vi "JY Mono Example.vi"() -> ()   [LabVIEW 2020]
doc: "This VI is an example on how to use the HORIBA Jobin Yvon Monochromator control VIs. To use this VI, press the Run button in LabVIEW.\n\nThe VI will retreive all configured monochromators from the computer's resgistry.\n\nSelect the desired monochromator from the Mono ID combo box and press the Connect button to start communications with that device. If the Force Initialization button is enabled, the monochromator will start its automatic calibration routine. If the Force Initialization button is not enabled, the sofwtare will keep the monochromator in its current positions.\n\nAfter connecting to the instrumnet, the VI will retreive the current positions of all movable motors in the system. This will continue until the Move To Target Position or Stop buttons are pressed.\n\nMove to Target Positions will move the monochromator to the postions entered in the indicators of the VI.\n\nStop will stop running the VI."
panel:
  out "Gratings":dbl[](array[numeric])=[1200.0, 300.0]
  in  "Target\nSide Exit":dbl
  in  "Target\nFront Exit":dbl
  in  "Target\nSide Entrance":dbl
  in  "Target\nFront Entrance":dbl
  in  "Exit Mirror":u16(ring)=2 caption="Target Position Exit Mirror" items=["Front"=2, "Side"=3]
  in  "Entrance Mirror":u16(ring)=2 caption="Target Position\nEntrance Mirror" items=["Front"=2, "Side"=3]
  out "error out":errorcluster
  in  "Target Grating":string(combo)="2"
  in  "Target WL":dbl=898.0
  in  "Move To\nTarget Positions":bool
  out "Units":string="nm"
  in  "Connect":bool
  out "Status":string="Initialized"
  out "Emulating":bool
  out "Initialized":bool=TRUE
  out "Current UniqueID":string="Mono4"
  in  "Force\nInitialization":bool
  in  "STOP":bool
  out "Units":string="mm"
  out "Units":string="mm"
  out "Units":string="mm"
  out "Units":string="mm"
  out "Side Exit":dbl
  out "Front Exit":dbl
  out "Side Entrance":dbl
  out "Front Entrance":dbl
  out "Exit Mirror\nPosition":i32(ring)=2 items=["EntranceMirror", "ExitMirror", "Front", "Side"]
  out "Entrance Mirror\nPosition":i32(ring)=2 items=["EntranceMirror", "ExitMirror", "Front", "Side"]
  out "Current Description":string="1" caption="Description"
  out "Grating Index":i32=1
  out "Current Grating":dbl=1200.0
  out "Current WL":dbl=897.9988
  in  "Mono ID":string(combo)="Mono4"
  # "Setup"
  # "Grating / Wavelength Control"
  # "Slits"
  # "Swing Mirrors"
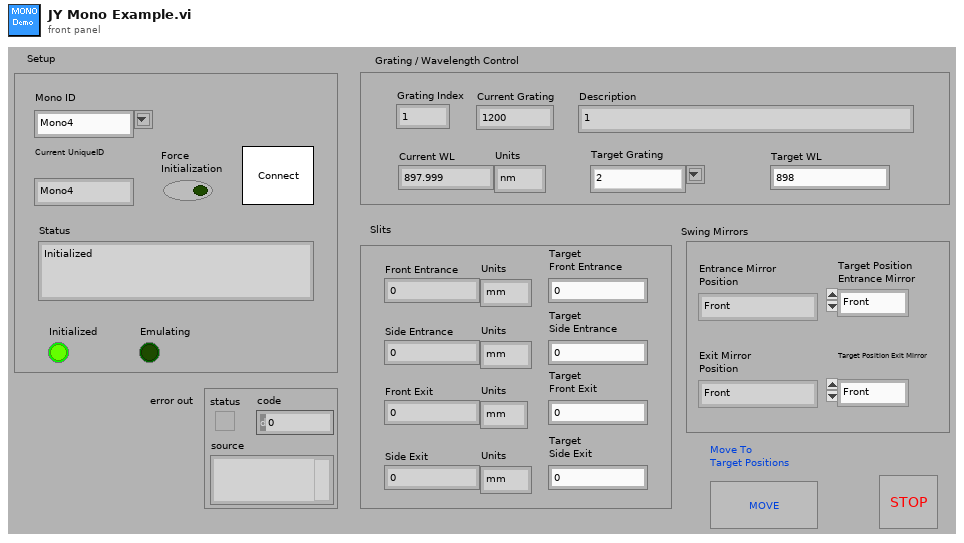
[diagram p1: front panel]
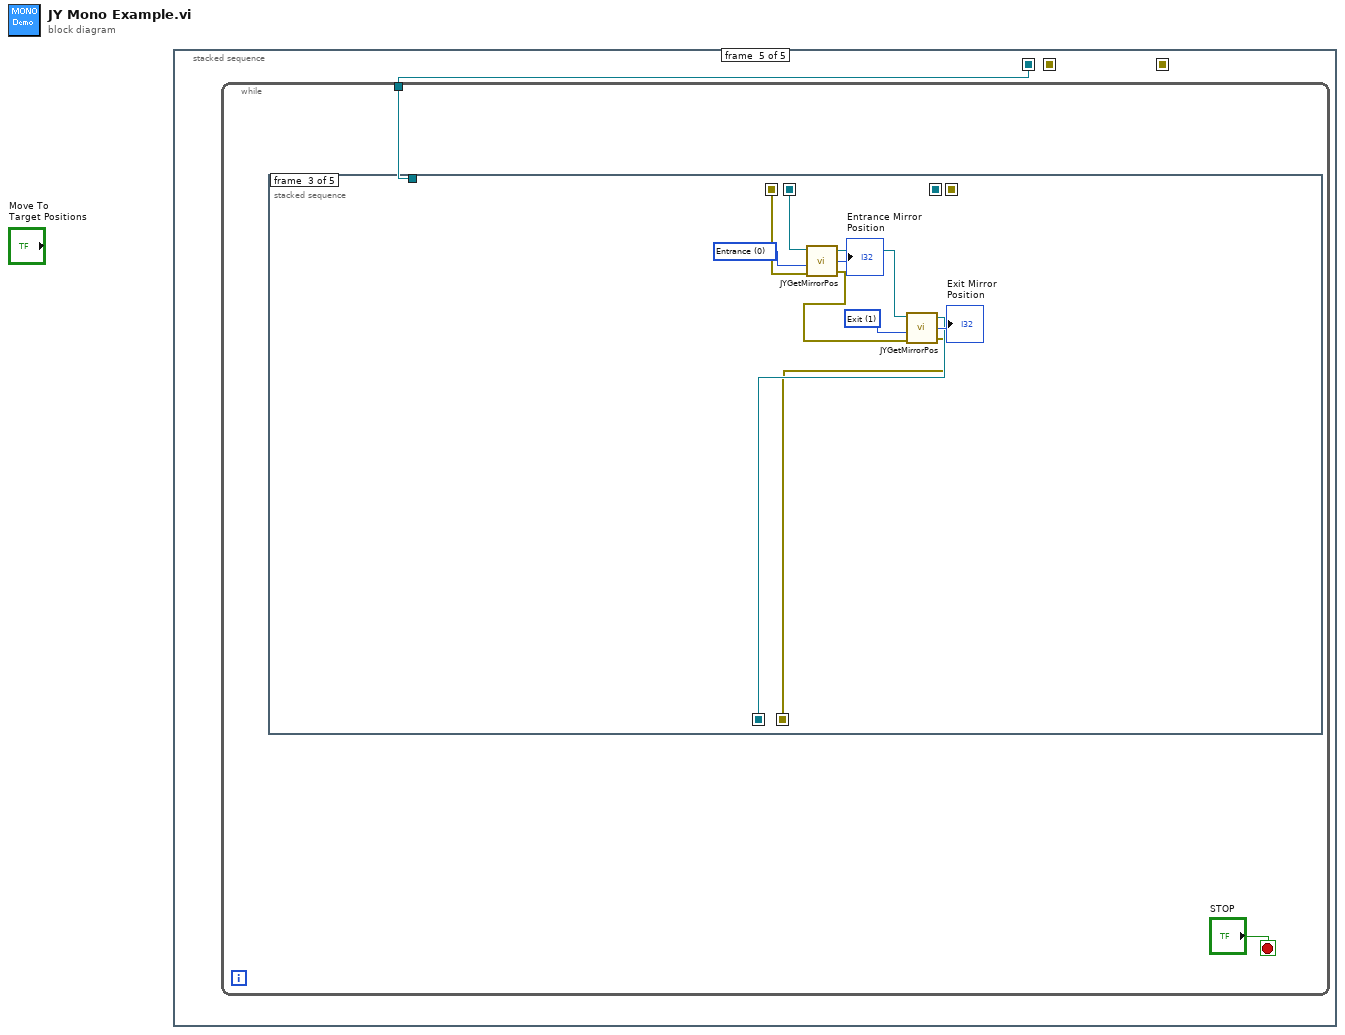
[diagram p0: block diagram]
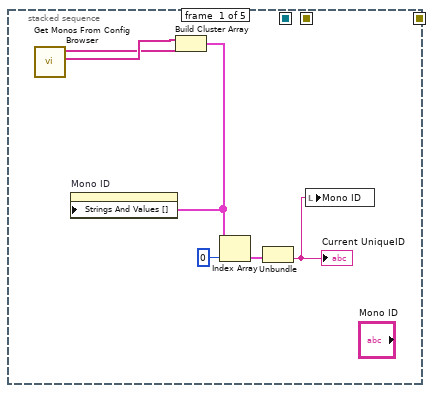
[diagram p2: hidden frame]
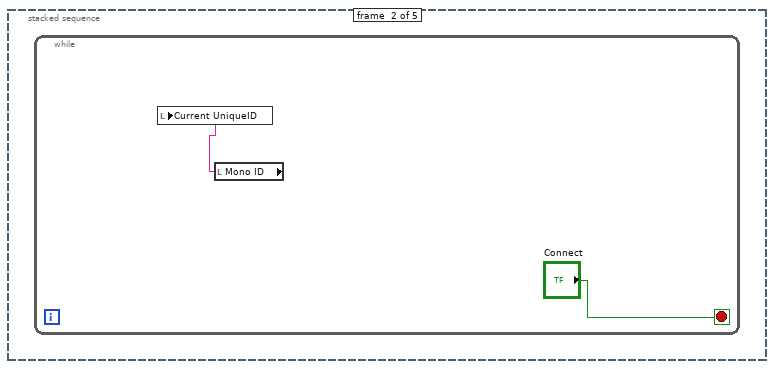
[diagram p3: hidden frame]
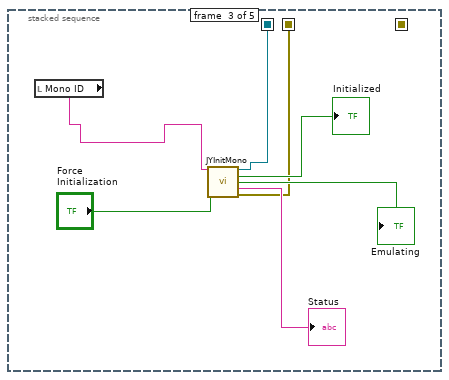
[diagram p4: hidden frame]
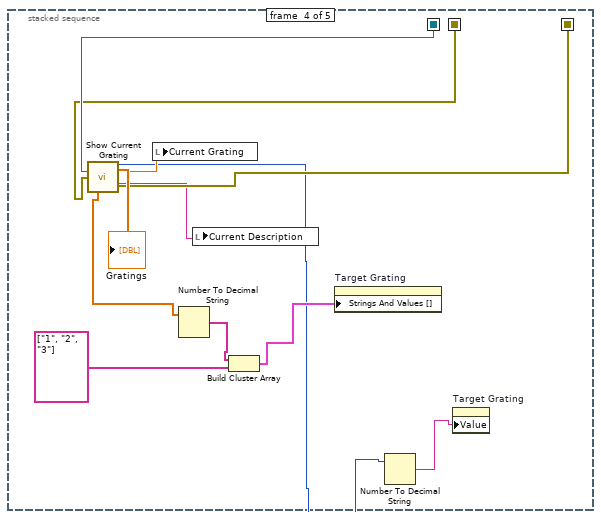
[diagram p5: hidden frame]
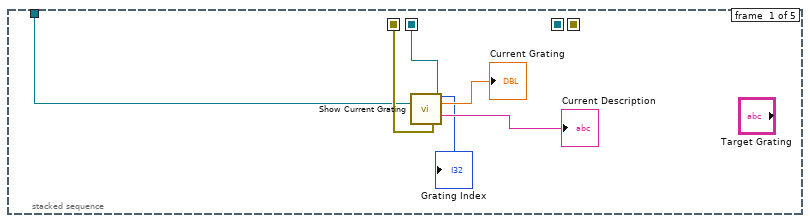
[diagram p6: hidden frame]
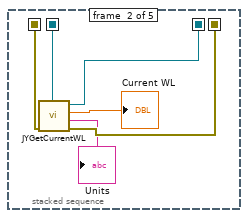
[diagram p7: hidden frame]
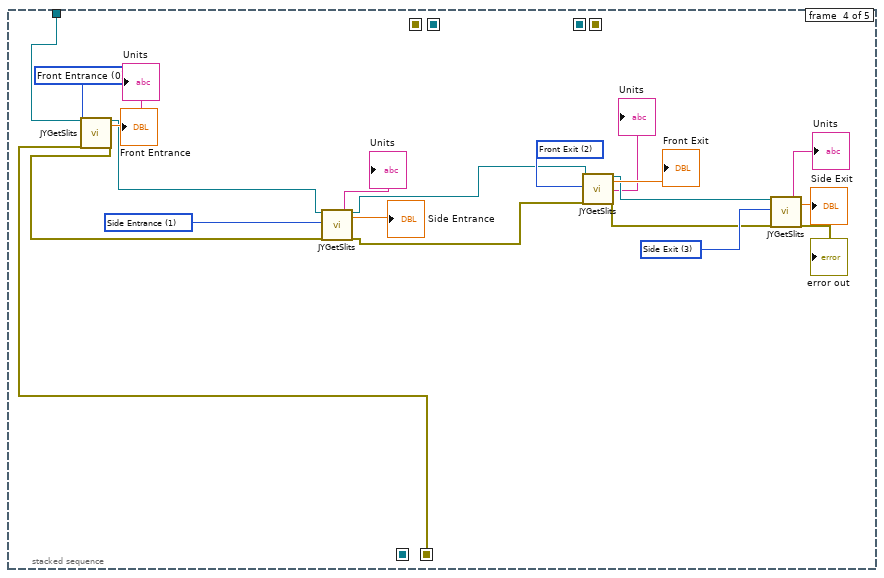
[diagram p8: hidden frame]
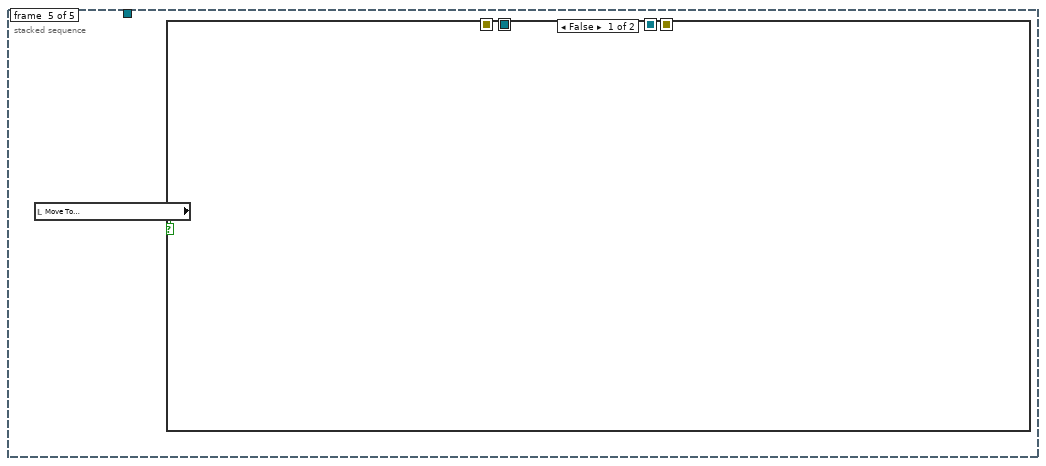
[diagram p9: hidden frame]
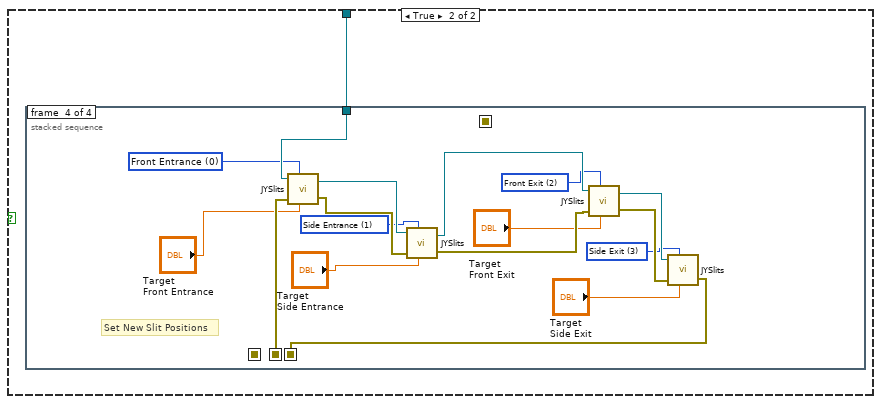
[diagram p10: hidden frame]
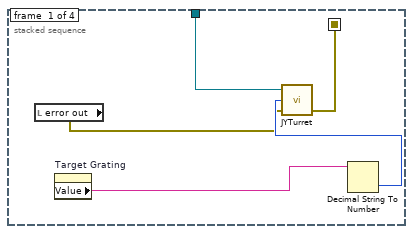
[diagram p11: hidden frame]
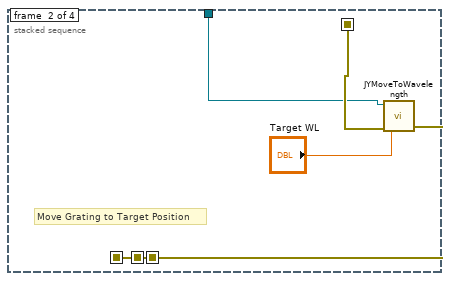
[diagram p12: hidden frame]
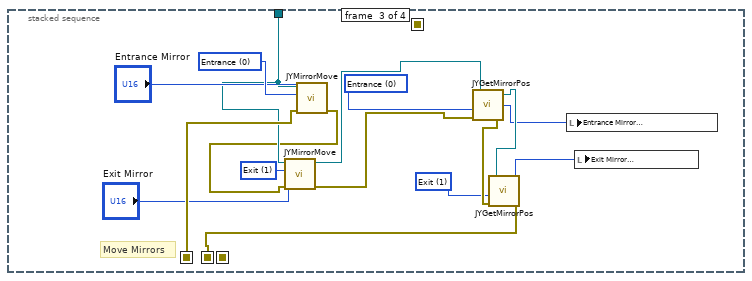
[diagram p13: hidden frame]
diagram:
  n1 = stacked-sequence {
    seq-local: [_ _ w10 _ _] -> [_ _ _ w22 w27]
    seq-local: [_ _ w9 _ _] -> [_ _ _ w21 _]
    seq-local: [_ _ _ w20 _] -> [_ _ _ _ _]
    frame #0 {
      n2 = call "Get Monos From Config Browser.vi"() -> ("UniqueIDs"=w5:string[], "Mono ID"=w6:string[])  [unwired: 3 in, 1 out]
      n3 = Build Cluster Array(w6, w5) -> (w3:cluster{"String":string, "String":string}[])
      n4 = property on="Mono ID" class="CmbBox"("Strings And Values []"=w3) -> ()  [unwired: 2 in, 2 out]
      n5 = Index Array(array=w3, index=0) -> (element=w4:cluster{"String":string, "String":string})
      n6 = Unbundle(w4) -> ("String"=w1:string)  [unwired: 1 out]
      "Current UniqueID" <- w1
      n7 = local write "Mono ID"(w1) -> ()
    }
    frame #1 {
      n8 = while {
        stop <- "Connect" stop-if-true
        n9 = local read "Mono ID"() -> (w7:string)
        n10 = local write "Current UniqueID"(w7) -> ()
      }
    }
    frame #2 {
      n11 = local read "Mono ID"() -> (w14:string)
      n12 = call "JYInitMono.vi"("Unique ID"=w14, "Force Init"="Force\nInitialization") -> ("Refnum out"=w10:refnum<k7>, "Initialized"=→"Initialized":bool, "Emulating"=→"Emulating":bool, "Status"=→"Status":string, "error out"=w9:errorcluster)  [unwired: 9 in]
    }
    frame #3 {
      n13 = call "Show Current Grating.vi"("Refnum in"=w22, "error in (no error)"=w21) -> ("Gratings"=w23:dbl[], "Grating Index"=w17:i32, "Current Grating"=w19:dbl, "Current Description"=w16:string, "error out"=w20:errorcluster)  [unwired: 5 in, 4 out]
      "Gratings" <- w23
      n14 = local write "Current Grating"(w19) -> ()
      n15 = Number To Decimal String(number=w23) -> (decimal integer string=w25:string[])  [unwired: 1 in]
      n16 = local write "Current Description"(w16) -> ()
      n17 = Build Cluster Array(w25, string[] ["1", "2", "3"]) -> (w26:cluster{"Numeric":string, string}[])
      n18 = property on="Target Grating" class="CmbBox"("Strings And Values []"=w26) -> ()  [unwired: 2 in, 2 out]
      n19 = Number To Decimal String(number=w17) -> (decimal integer string=w18:string)  [unwired: 1 in]
      n20 = property on="Target Grating" class="CmbBox"("Value"=w18) -> ()  [unwired: 2 in, 2 out]
    }
    frame #4 {
      n21 = while {
        tunnel: w27 -> [w28]
        stop <- "STOP" stop-if-true
        n22 = stacked-sequence {
          seq-local: [w33 _ _ _ _] -> [_ w40 w51 _ w73]
          seq-local: [w32 _ _ _ _] -> [_ w39 w50 _ _]
          seq-local: [_ w38 _ _ _] -> [_ _ _ _ _]
          seq-local: [_ w37 _ _ _] -> [_ _ _ _ _]
          seq-local: [_ _ w43 _ _] -> [_ _ _ _ _]
          seq-local: [_ _ w42 _ _] -> [_ _ _ w52 _]
          tunnel: w28 -> [w31 _ _ w53 _]
          frame #0 {
            n23 = call "Show Current Grating.vi"("Refnum in"=w31) -> ("Grating Index"=→"Grating Index":i32, "Current Grating"=→"Current Grating":dbl, "Current Description"=→"Current Description":string, "error out"=w32:errorcluster, "JYMONOLib.IJYMonoReqd"=w33:refnum<k7>)  [unwired: 6 in, 4 out]
          }
          frame #1 {
            n24 = call "JYGetCurrentWL.vi"("error in (no error)"=w39, "JYMONOLib.IJYMonoReqd"=w40) -> ("error out"=w37:errorcluster, "Units"=→"Units":string, "Current WL"=→"Current WL":dbl, "JYMONOLib.IJYMonoReqd 2"=w38:refnum<k7>)  [unwired: 6 in]
          }
          frame #2 {
            w48 = u16 1 items=["Entrance", "Exit"] ("Mirror Number")
            w49 = u16 0 items=["Entrance", "Exit"] ("Mirror Number")
            n25 = call "JYGetMirrorPos.vi"("error in (no error)"=w50, "Mirror"=w49, "Refnum In"=w51) -> ("error out"=w46:errorcluster, "Current Mirror Position"=→"Entrance Mirror\nPosition":i32, "Refnum Out"=w47:refnum<k7>)  [unwired: 1 in]
            n26 = call "JYGetMirrorPos.vi"("error in (no error)"=w46, "Mirror"=w48, "Refnum In"=w47) -> ("error out"=w42:errorcluster, "Current Mirror Position"=→"Exit Mirror\nPosition":i32, "Refnum Out"=w43:refnum<k7>)  [unwired: 1 in]
          }
          frame #3 {
            w65 = u16 3 items=["Front Entrance", "Side Entrance", "Front Exit", "Side Exit", "First Intermediate", "Second Intermediate"] ("Slit")
            w66 = u16 2 items=["Front Entrance", "Side Entrance", "Front Exit", "Side Exit", "First Intermediate", "Second Intermediate"] ("Slit")
            w67 = u16 1 items=["Front Entrance", "Side Entrance", "Front Exit", "Side Exit", "First Intermediate", "Second Intermediate"] ("Slit")
            w68 = u16 0 items=["Front Entrance", "Side Entrance", "Front Exit", "Side Exit", "First Intermediate", "Second Intermediate"] ("Slit")
            n27 = call "JYGetSlits.vi"("MonoRefNum IN"=w53, "Slit"=w68, "error in (no error)"=w52) -> ("Units"=→"Units":string, "MonoRefNum Out"=w64:refnum<k7>, "Slit Width"=→"Front Entrance":dbl, "error out"=w61:errorcluster)  [unwired: 13 in]
            n28 = call "JYGetSlits.vi"("MonoRefNum IN"=w64, "Slit"=w67, "error in (no error)"=w61) -> ("Units"=→"Units":string, "MonoRefNum Out"=w63:refnum<k7>, "Slit Width"=→"Side Entrance":dbl, "error out"=w60:errorcluster)  [unwired: 13 in]
            n29 = call "JYGetSlits.vi"("MonoRefNum IN"=w63, "Slit"=w66, "error in (no error)"=w60) -> ("Units"=→"Units":string, "MonoRefNum Out"=w62:refnum<k7>, "Slit Width"=→"Front Exit":dbl, "error out"=w59:errorcluster)  [unwired: 13 in]
            n30 = call "JYGetSlits.vi"("MonoRefNum IN"=w62, "Slit"=w65, "error in (no error)"=w59) -> ("Units"=→"Units":string, "Slit Width"=→"Side Exit":dbl, "error out"=→"error out":errorcluster)  [unwired: 13 in, 1 out]
          }
          frame #4 {
            n31 = local read "Move To\nTarget Positions"() -> (w74:bool)
            n32 = case shown="False" w74 {
              tunnel: w73 -> [_ w75]
              frame False {
              }
              frame True {
                n33 = stacked-sequence {
                  seq-local: [w77 _ _ _] -> [_ w83 _ _]
                  seq-local: [_ w81 _ _] -> [_ _ w98 _]
                  seq-local: [_ _ w85 _] -> [_ _ _ w116]
                  seq-local: [_ _ _ w109] -> [_ _ _ _]
                  tunnel: w75 -> [w79 w82 w96 w117]
                  frame #0 {
                    n34 = local read "error out"() -> (w78:errorcluster)
                    n35 = property on="Target Grating" class="CmbBox"() -> ("Value"=w76:string)  [unwired: 2 in, 2 out]
                    n36 = Decimal String To Number(string=w76) -> (number=w80:i32)  [unwired: 2 in, 1 out]
                    n37 = call "JYTurret.vi"("error in (no error)"=w78, "Grating Index"=w80, "JYMONOLib.IJYMonoReqd"=w79) -> ("error out"=w77:errorcluster)  [unwired: 2 out]
                  }
                  frame #1 {
                    # "Move Grating to Target Position"
                    n38 = call "JYMoveToWavelength.vi"("error in (no error)"=w83, "Target WL"="Target WL", "RefNum In"=w82) -> ("error out"=w81:errorcluster)  [unwired: 1 in, 2 out]
                  }
                  frame #2 {
                    w91 = u16 1 items=["Entrance", "Exit"] ("Mirror Number")
                    w90 = u16 0 items=["Entrance", "Exit"] ("Mirror Number")
                    w97 = u16 1 items=["Entrance", "Exit", "Front", "Side"] ("Mirror Number")
                    w100 = u16 0 items=["Entrance", "Exit", "Front", "Side"] ("Mirror Number")
                    # "Move Mirrors"
                    n39 = call "JYMirrorMove.vi"("error in (no error)"=w98, "Mirror Position"="Entrance Mirror", "Mirror Number"=w100, "RefNum In"=w96) -> ("error out"=w95:errorcluster)  [unwired: 6 in, 1 out]
                    n40 = call "JYMirrorMove.vi"("error in (no error)"=w95, "Mirror Position"="Exit Mirror", "Mirror Number"=w97, "RefNum In"=w96) -> ("error out"=w88:errorcluster, "MonoRefNum Out"=w89:refnum<k7>)  [unwired: 6 in]
                    n41 = call "JYGetMirrorPos.vi"("error in (no error)"=w88, "Mirror"=w90, "Refnum In"=w89) -> ("error out"=w93:errorcluster, "Current Mirror Position"=w87:i32, "Refnum Out"=w92:refnum<k7>)  [unwired: 1 in]
                    n42 = call "JYGetMirrorPos.vi"("error in (no error)"=w93, "Mirror"=w91, "Refnum In"=w92) -> ("error out"=w85:errorcluster, "Current Mirror Position"=w86:i32)  [unwired: 1 in, 1 out]
                    n43 = local write "Entrance Mirror\nPosition"(w87) -> ()
                    n44 = local write "Exit Mirror\nPosition"(w86) -> ()
                  }
                  frame #3 {
                    w102 = u16 3 items=["Front Entrance", "Side Entrance", "Front Exit", "Side Exit", "First Intermediate", "Second Intermediate"] ("Slit")
                    w104 = u16 2 items=["Front Entrance", "Side Entrance", "Front Exit", "Side Exit", "First Intermediate", "Second Intermediate"] ("Slit")
                    w106 = u16 1 items=["Front Entrance", "Side Entrance", "Front Exit", "Side Exit", "First Intermediate", "Second Intermediate"] ("Slit")
                    w108 = u16 0 items=["Front Entrance", "Side Entrance", "Front Exit", "Side Exit", "First Intermediate", "Second Intermediate"] ("Slit")
                    # "Set New Slit Positions"
                    n45 = call "JYSlits.vi"("JYMONOLib.IJYMonoReqd"=w117, "Slit"=w108, "error in (no error)"=w116, "Slit Width"="Target\nFront Entrance") -> ("JYMONOLib.IJYMonoReqd 2"=w115:refnum<k7>, "error out"=w112:errorcluster)  [unwired: 1 in]
                    n46 = call "JYSlits.vi"("JYMONOLib.IJYMonoReqd"=w115, "Slit"=w106, "error in (no error)"=w112, "Slit Width"="Target\nSide Entrance") -> ("JYMONOLib.IJYMonoReqd 2"=w114:refnum<k7>, "error out"=w111:errorcluster)  [unwired: 1 in]
                    n47 = call "JYSlits.vi"("JYMONOLib.IJYMonoReqd"=w114, "Slit"=w104, "error in (no error)"=w111, "Slit Width"="Target\nFront Exit") -> ("JYMONOLib.IJYMonoReqd 2"=w113:refnum<k7>, "error out"=w110:errorcluster)  [unwired: 1 in]
                    n48 = call "JYSlits.vi"("JYMONOLib.IJYMonoReqd"=w113, "Slit"=w102, "error in (no error)"=w110, "Slit Width"="Target\nSide Exit") -> ("error out"=w109:errorcluster)  [unwired: 1 in, 1 out]
                  }
                }
              }
            }
          }
        }
      }
    }
  }
